vi "ask.vi"() -> ()   [LabVIEW 2014]
uses:
  <vilib>/Analysis/NI_AALPro.lvlib
panel:
  out "dig.data":dbl[](graph)
  out "demod":dynamicdata(graph)
  out "modulated":dynamicdata(graph)
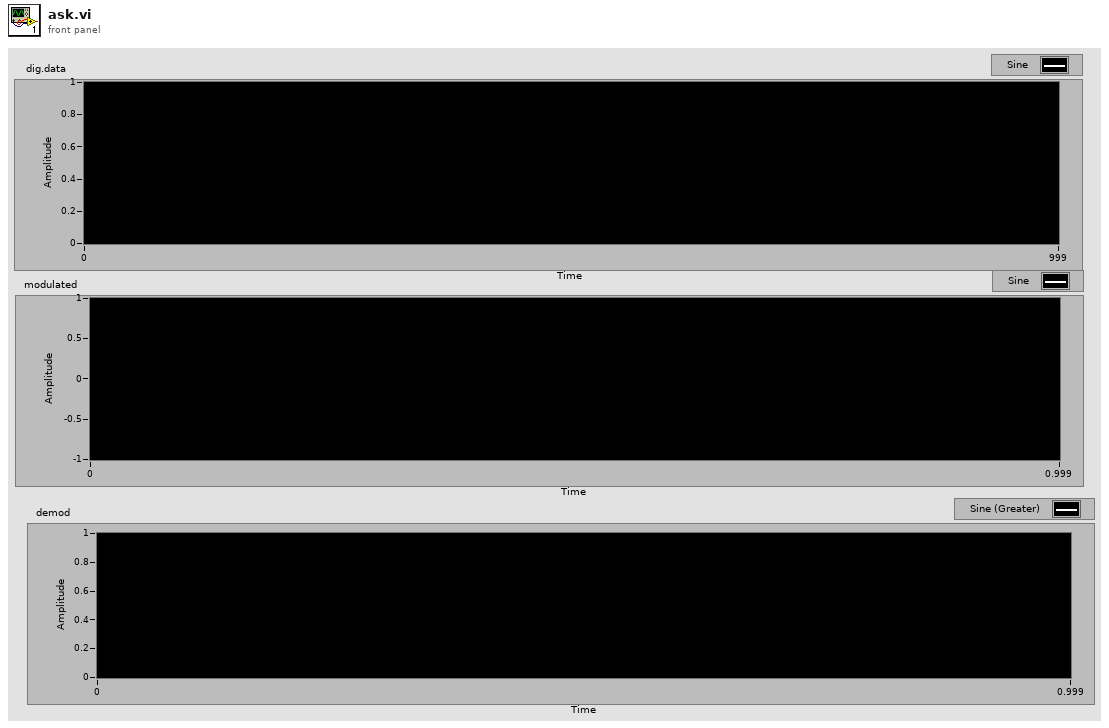
[diagram p1: front panel]
types:
  T1 = enum16{"sine", "cosine", "triangle", "square", "sawtooth", "increasing ramp", "decreasing ramp"}
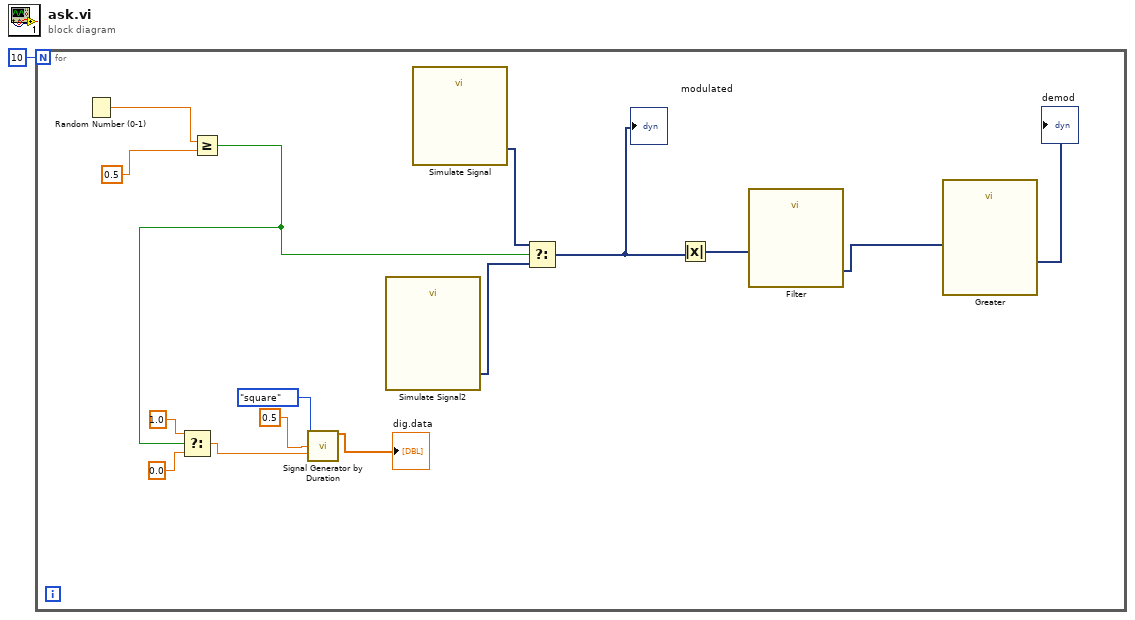
[diagram p0: block diagram]
diagram:
  n1 = for {
    N: 10 -> [_]
    n2 = Random Number (0-1)() -> (number: 0 to 1=w14:dbl)
    n3 = Greater Or Equal?(x=w14, y=0.5) -> (x >= y?=w8:bool)
    n4 = Select(t=1.0, s=w8, f=0.0) -> (s? t:f=w5:dbl)
    n5 = call <vilib>:"Signal Generator by Duration.vi"("signal type"=T1."square", "frequency"=0.5, "amplitude"=w5) -> ("signal"=→"dig.data":dbl[])  [unwired: 9 in, 3 out]
    n6 = call "Simulate Signal2"() -> ("Sine"=w12:dynamicdata)  [unwired: 14 in, 1 out]
    n7 = call "Simulate Signal"() -> ("Sine"=w13:dynamicdata)  [unwired: 14 in, 1 out]
    n8 = Select(t=w13, s=w8, f=w12) -> (s? t:f=w11:dynamicdata)
    "modulated" <- w11
    n9 = Absolute Value(x=w11) -> (abs(x)=w16:dynamicdata)
    n10 = call "Filter"("Signal"=w16) -> ("Filtered Signal"=w10:dynamicdata)  [unwired: 9 in, 1 out]
    n11 = call "Greater"("Operand 1"=w10) -> ("Result"=→"demod":dynamicdata)  [unwired: 9 in, 1 out]
  }
